vi "Ex1-Check-file.vi"() -> ()   [LabVIEW 2021]
panel:
  in  "file path (use dialog)":path
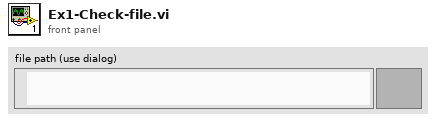
[diagram p1: front panel]
types:
  T1 = enum16{"open", "replace", "create", "open or create", "replace or create", "replace or create with confirmation"}
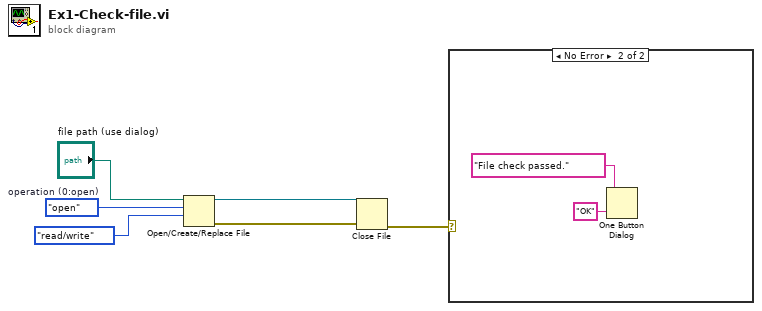
[diagram p0: block diagram]
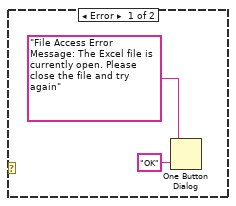
[diagram p2: hidden frame]
diagram:
  w3 = T1."open"  # operation (0:open)
  n1 = Open/Create/Replace File(file path (use dialog)="file path (use dialog)", operation (0:open)=w3, access (0:read/write)=enum16{"read/write", "read-only", "write-only"}."read/write") -> (refnum out=w6:refnum<file>, error out=w5:errorcluster)  [unwired: 3 in, 1 out]
  n2 = Close File(refnum=w6, error in=w5) -> (error out=w1:errorcluster)  [unwired: 1 out]
  n3 = case shown="No Error" w1 {
    frame Error {
      n4 = One Button Dialog(message="File Access Error Message: The Excel file is currently open. Please close the file and try again", button name ("OK")="OK") -> ()  [unwired: 1 out]
    }
    frame No Error {
      n5 = One Button Dialog(message="File check passed.", button name ("OK")="OK") -> ()  [unwired: 1 out]
    }
  }
